vi "初始化数据库.vi"(8 "error in (no error)":errorcluster, 11 "ADODB._Connection In":refnum<k7>) -> (0 "error out":errorcluster)   [LabVIEW 2015]
uses:
  Database_util/Ctl/DNS.ctl
  Database_util/Ctl/database_Method.ctl
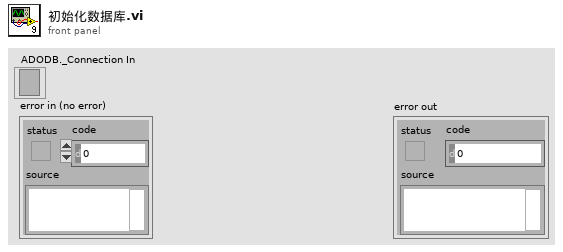
[diagram p1: front panel]
types:
  T1 = typedef "database_Method.ctl" = enum16{"初始化", "查询", "关闭"}
  T2 = typedef "DNS.ctl" = string
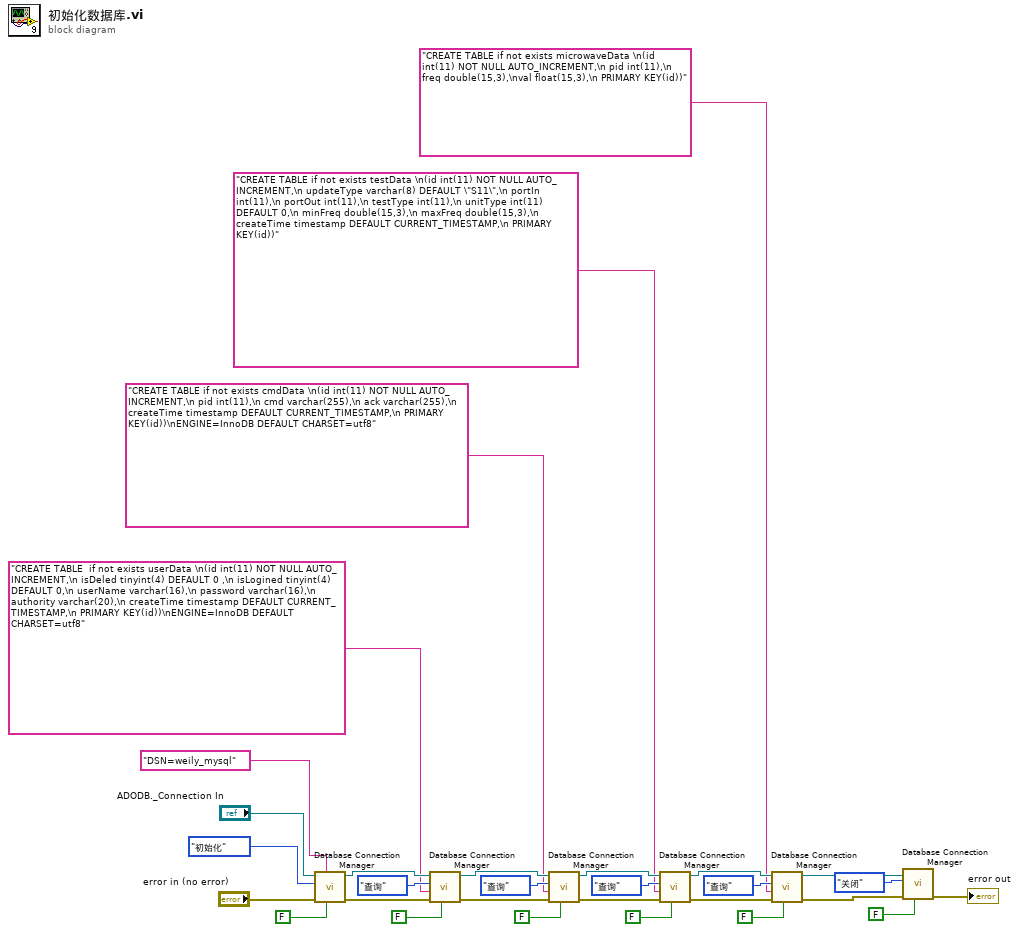
[diagram p0: block diagram]
diagram:
  n1 = call "Database Connection Manager.vi"("Return Data (T)"=FALSE, "ConnectionString"=T2 "DSN=weily_mysql", "error in (no error)"="error in (no error)", "Method"=database_Method."初始化", "ADODB._Connection In"="ADODB._Connection In") -> ("error out"=w24:errorcluster, "ADODB._Connection Out"=w25:refnum<k7>)  [unwired: 3 in, 2 out]
  n2 = call "Database Connection Manager.vi"("Return Data (T)"=FALSE, "error in (no error)"=w24, "Command Text"="CREATE TABLE  if not exists userData \n(id int(11) NOT NULL AUTO_INCREMENT,\n isDeled tinyint(4) DEFAULT 0 ,\n isLogined tinyint(4) DEFAULT 0,\n userName varchar(16),\n password varchar(16),\n authority varchar(20),\n createTime timestamp DEFAULT CURRENT_TIMESTAMP,\n PRIMARY KEY(id))\nENGINE=InnoDB DEFAULT CHARSET=utf8", "Method"=database_Method."查询", "ADODB._Connection In"=w25) -> ("error out"=w19:errorcluster, "ADODB._Connection Out"=w20:refnum<k7>)  [unwired: 3 in, 2 out]
  n3 = call "Database Connection Manager.vi"("Return Data (T)"=FALSE, "error in (no error)"=w19, "Command Text"="CREATE TABLE if not exists cmdData \n(id int(11) NOT NULL AUTO_INCREMENT,\n pid int(11),\n cmd varchar(255),\n ack varchar(255),\n createTime timestamp DEFAULT CURRENT_TIMESTAMP,\n PRIMARY KEY(id))\nENGINE=InnoDB DEFAULT CHARSET=utf8" ("SQL"), "Method"=database_Method."查询", "ADODB._Connection In"=w20) -> ("error out"=w15:errorcluster, "ADODB._Connection Out"=w16:refnum<k7>)  [unwired: 3 in, 2 out]
  n4 = call "Database Connection Manager.vi"("Return Data (T)"=FALSE, "error in (no error)"=w15, "Command Text"="CREATE TABLE if not exists testData \n(id int(11) NOT NULL AUTO_INCREMENT,\n updateType varchar(8) DEFAULT \"S11\",\n portIn int(11),\n portOut int(11),\n testType int(11),\n unitType int(11) DEFAULT 0,\n minFreq double(15,3),\n maxFreq double(15,3),\n createTime timestamp DEFAULT CURRENT_TIMESTAMP,\n PRIMARY KEY(id))" ("SQL"), "Method"=database_Method."查询", "ADODB._Connection In"=w16) -> ("error out"=w11:errorcluster, "ADODB._Connection Out"=w12:refnum<k7>)  [unwired: 3 in, 2 out]
  n5 = call "Database Connection Manager.vi"("Return Data (T)"=FALSE, "error in (no error)"=w11, "Command Text"="CREATE TABLE if not exists microwaveData \n(id int(11) NOT NULL AUTO_INCREMENT,\n pid int(11),\n freq double(15,3),\nval float(15,3),\n PRIMARY KEY(id))" ("SQL"), "Method"=database_Method."查询", "ADODB._Connection In"=w12) -> ("error out"=w2:errorcluster, "ADODB._Connection Out"=w3:refnum<k7>)  [unwired: 3 in, 2 out]
  n6 = call "Database Connection Manager.vi"("Return Data (T)"=FALSE, "error in (no error)"=w2, "Method"=database_Method."关闭", "ADODB._Connection In"=w3) -> ("error out"=→"error out":errorcluster)  [unwired: 4 in, 3 out]
